vi "snap_usrp_tx.vi"() -> ()   [LabVIEW 2014]
uses:
  <vilib>/userdefined/High Color/IMAQdx.ctl
  <vilib>/vision/driver/IMAQdx.llb/IMAQdx Camera Control Mode.ctl
  <vilib>/addons/Modulation/Analog/support/mod_Set Error Source.vi
  var_stop.vi
  <vilib>/addons/Modulation/Digital/Support/Common/Validators/mod_Generate Filter Coefficients Validate.vi
  <vilib>/addons/Modulation/Digital/General/subVIs/mod_Generate Filter Coefficients.vi
  <vilib>/addons/Modulation/Digital/General/MT Apply Pulse Shaping Filter (Generic).vi
  <instrlib>/niUSRP/niUSRP Write Tx Data (CDB Cluster).vi
  <vilib>/vision/driver/NI_Vision_Acquisition_Software.lvlib
  <resource>/objmgr/imaqdx.rc
  <vilib>/addons/Modulation/niDMT.lvlib
panel:
  in  "type":enum16{"binary", "quadrature"}(ring)
  out "error IO":errorcluster
  in  "bytes per packet":i32
  in  "millisecond multiple":u32
  in  "stop":bool
  in  "Quality (750)":i32=750
  in  "Compression (None)":i32(ring) items=["None", "JPEG", "PACKED BINARY"]
  out "Image":T1(plugin-control)
  in  "Clocking and Synchronization:Timebase Clock Source":string(combo)="Internal"
  in  "Clocking and Synchronization:Reference Frequency Source":string(combo)="Internal"
  in  "Active Channel":string
  out "coerced gain":dbl format="%#_6f"
  out "coerced carrier frequency":dbl=100000.0 format="%#_6p"
  out "coerced IQ rate":dbl=100000.0 format="%#_6p"
  in  "active antenna":string
  in  "gain":dbl format="%#_6f"
  in  "carrier frequency":dbl=100000.0 format="%#_6p"
  in  "IQ rate":dbl=100000.0 format="%#_6p"
  in  "device names":refnum<k15>
  in  "VideoMode":u32
  in  "Camera Control Mode":T2
  in  "Session In":T3
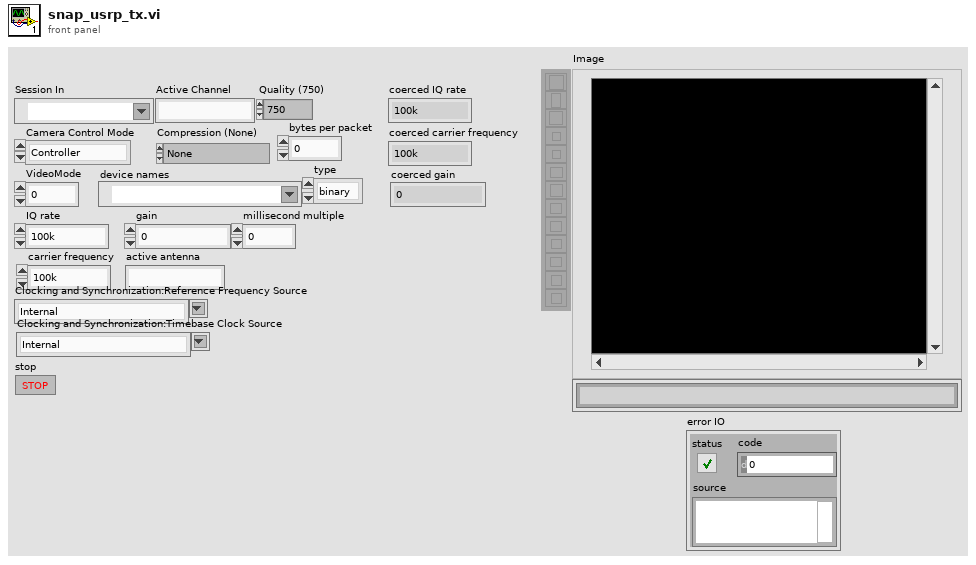
[diagram p1: front panel]
types:
  T1 = typedef "IMAQ Image.ctl" = refnum<image>
  T2 = typedef "NI_Vision_Acquisition_Software.lvlib/IMAQdx Camera Control Mode.ctl" = enum32{"Controller", "Listener"}
  T3 = typedef "IMAQdx.ctl" = refnum<k21>
  T4 = enum16{"none", "Raised Cosine", "Root Raised Cos", "Gaussian"}
  T5 = enum16{"FSK", "PSK", "QAM", "MSK", "PAM", "ASK", "CPM"}
  T6 = typedef "niAMT.lvlib/Complex Data Waveform.ctl" = cluster{"t0":dbl, "dt":dbl, "Y":cdb[]}
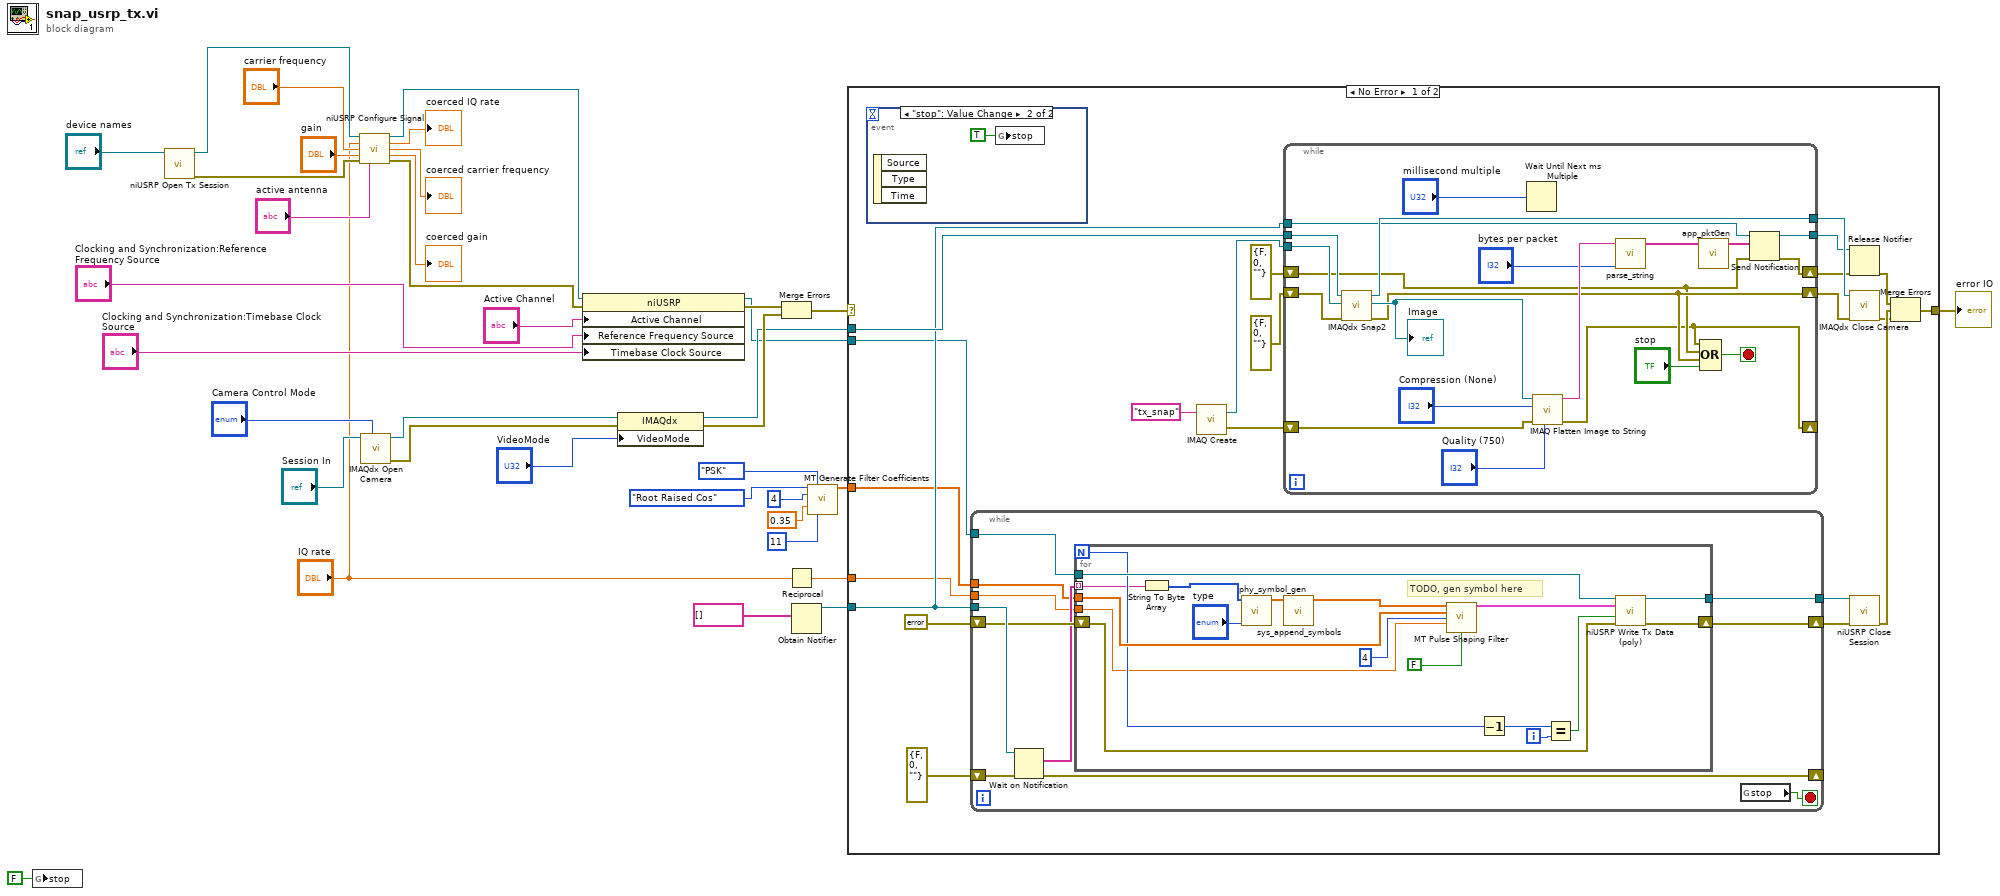
[diagram p0: block diagram]
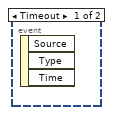
[diagram p2: hidden frame]
diagram:
  n1 = global write "var_stop.vi" "stop"(FALSE) -> ()
  n2 = call <instrlib>:"niUSRP Open Tx Session.vi"("device names"="device names") -> ("session handle out"=w31:refnum<k15>, "error out"=w29:errorcluster)  [unwired: 13 in]
  n3 = call <instrlib>:"niUSRP Configure Signal.vi"("session handle"=w31, "IQ rate"="IQ rate", "carrier frequency"="carrier frequency", "gain"="gain", "error in (no error)"=w29, "active antenna"="active antenna") -> ("session handle out"=w25:refnum<k15>, "coerced IQ rate"=→"coerced IQ rate":dbl, "coerced carrier frequency"=→"coerced carrier frequency":dbl, "coerced gain"=→"coerced gain":dbl, "error out"=w24:errorcluster)  [unwired: 5 in]
  n4 = call <vilib>:"IMAQdx Open Camera.vi"("Camera Control Mode"="Camera Control Mode", "Session In"="Session In") -> ("error out"=w33:errorcluster, "Session Out"=w34:T3)  [unwired: 8 in]
  n5 = property class="niUSRP"(reference=w25, error in=w24, "Active Channel"="Active Channel", "Reference Frequency Source"="Clocking and Synchronization:Reference Frequency Source", "Timebase Clock Source"="Clocking and Synchronization:Timebase Clock Source") -> (reference out=w10:refnum<k15>, error out=w17:errorcluster)
  n6 = property class="IMAQdx"(reference=w34, error in=w33, "VideoMode"="VideoMode") -> (reference out=w14:T3, error out=w16:errorcluster)
  n7 = Merge Errors(w17, w16) -> (w15:errorcluster)
  n8 = Reciprocal(x="IQ rate") -> (1/x=w1:dbl)
  n9 = Obtain Notifier(notification data type=string[] [] ("packets")) -> (notifier out=w12:refnum<notifier>)  [unwired: 3 in, 2 out]
  n10 = call <vilib>:"MT Generate Filter Coefficients.vi"("pulse shaping filter (none)"=T4."Root Raised Cos", "modulation type"=T5."PSK", "pulse shaping samples per symbol (16)"=4, "filter parameter"=0.35, "filter length (symbols)"=11) -> ("pulse shaping filter coefficients"=w3:dbl[])  [unwired: 8 in, 2 out]
  n11 = case shown="No Error" w15 {
    selector: w15 -> [_ w110]
    tunnel: w14 -> [w56 _]
    tunnel: w12 -> [w51 _]
    tunnel: w10 -> [w48 _]
    tunnel: [w41 w110] -> w9
    tunnel: w3 -> [w40 _]
    tunnel: w1 -> [w39 _]
    frame No Error {
      n12 = event shown="[1] \"stop\": Value Change" {
        selector: _ -> [_ _]
        dyn-events: _ -> [_ _]
        timeout: _ -> [_ _]
        event Timeout {
          n13 = event-data() -> ()  [unwired: 1 in, 3 out]
        }
        event "stop": Value Change {
          n14 = event-data() -> ()  [unwired: 1 in, 3 out]
          n15 = global write "var_stop.vi" "stop"(TRUE) -> ()
        }
      }
      n16 = while {
        shift-right: [w89] -> w53
        shift-left: errorcluster {"status"=FALSE, "code"=0, "source"=""} ("error out") -> [w85]
        tunnel: w51 -> [w88]
        shift-right: [w87] -> _
        shift-left: errorcluster {"status"=FALSE, "code"=0, "source"=""} ("error out") -> [w86]
        tunnel: [w84] -> w49
        tunnel: w48 -> [w83]
        tunnel: w40 -> [w81]
        tunnel: w39 -> [w80]
        stop <- w90 stop-if-true
        n17 = Wait on Notification(notifier=w88, error in (no error)=w86) -> (notification=w82:string[], error out=w87:errorcluster)  [unwired: 2 in, 2 out]
        n18 = for {
          N -> [w99]
          shift-right: [w108] -> w89
          shift-left: w85 -> [w107]
          tunnel: [w106] -> w84
          tunnel: w83 -> [w105]
          tunnel: w82 -> [w96] mode=indexing
          tunnel: w81 -> [w104]
          tunnel: w80 -> [w93]
          i -> [w100]
          # "TODO, gen symbol here"
          n19 = String To Byte Array(string=w96) -> (unsigned byte array=w95:u8[])
          n20 = call "phy_symbol_gen.vi"("type"="type", "Input bytes"=w95) -> ("symbols"=w92:cdb[])  [unwired: 9 in]
          n21 = call "sys_append_symbols.vi"("raw symbols"=w92) -> ("appended symbols"=w91:cdb[])  [unwired: 10 in]
          n22 = call-poly <vilib>:"MT Pulse Shaping Filter.vi"("symbols"=w91, "pulse shaping filter coefficients"=w104, "samples per symbol (16)"=4, "symbol rate (Hz)"=w93, "reset? (T)"=FALSE) -> ("output complex waveform"=w101:T6)  [unwired: 9 in, 1 out]
          n23 = Decrement(x=w99) -> (x-1=w98:i32)
          n24 = Equal?(x=w98, y=w100) -> (x = y?=w97:bool)
          n25 = call-poly <instrlib>:"niUSRP Write Tx Data (poly).vi"("session handle"=w105, "data"=w101, "end of data?"=w97, "error in (no error)"=w107) -> ("session handle out"=w106:refnum<k15>, "error out"=w108:errorcluster)  [unwired: 10 in]
        }
        n26 = global read "var_stop.vi" "stop"() -> (w90:bool)
      }
      n27 = call "IMAQ Create"("Image Name"="tx_snap") -> ("New Image"=w57:T1, "error out"=w45:errorcluster)  [unwired: 4 in]
      n28 = while {
        tunnel: w57 -> [w79]
        tunnel: w56 -> [w78]
        shift-right: [w64] -> w54
        shift-left: errorcluster {"status"=FALSE, "code"=0, "source"=""} ("error out") -> [w77]
        tunnel: [w76] -> w55
        tunnel: w51 -> [w72]
        shift-right: [w66] -> w38
        shift-left: errorcluster {"status"=FALSE, "code"=0, "source"=""} ("error out") -> [w63]
        shift-right: [w60] -> _
        shift-left: w45 -> [w61]
        tunnel: [w59] -> w37
        stop <- w62 stop-if-true
        n29 = call <vilib>:"IMAQdx Snap2.vi"("error in"=w77, "Image In"=w79, "Session In"=w78) -> ("error out"=w64:errorcluster, "Image Out"=w75:T1, "Session Out"=w76:T3)  [unwired: 6 in]
        "Image" <- w75
        n30 = Wait Until Next ms Multiple(millisecond multiple="millisecond multiple") -> ()  [unwired: 1 out]
        n31 = call "IMAQ Flatten Image to String"("Quality (750)"="Quality (750)", "error in (no error)"=w61, "Compression (None)"="Compression (None)", "Image"=w75) -> ("error out"=w60:errorcluster, "Data String"=w70:string)  [unwired: 6 in]
        n32 = call "parse_string.vi"("bytes per packet"="bytes per packet", "original content"=w70) -> ("appended array"=w68:string[])  [unwired: 9 in]
        n33 = call "app_pktGen.vi"("appended array"=w68) -> ("packets"=w67:string[])  [unwired: 10 in]
        n34 = Compound Arithmetic op=OR(w60, w63, w64, "stop") -> (w62:bool)
        n35 = Send Notification(notification=w67, notifier=w72, error in (no error)=w63) -> (notifier out=w59:refnum<notifier>, error out=w66:errorcluster)
      }
      n36 = Release Notifier(notifier=w37, error in (no error)=w38) -> (error out=w44:errorcluster)  [unwired: 1 in, 2 out]
      n37 = call <vilib>:"IMAQdx Close Camera.vi"("error in"=w54, "Session In"=w55) -> ("error out"=w42:errorcluster)  [unwired: 9 in]
      n38 = call <instrlib>:"niUSRP Close Session.vi"("session handle"=w49, "error in (no error)"=w53) -> ("error out"=w43:errorcluster)  [unwired: 13 in]
      n39 = Merge Errors(w44, w43, w42) -> (w41:errorcluster)
    }
    frame Error {
    }
  }
  "error IO" <- w9
